vi "Coord window-Generate picture.vi"(8 "error in (no error)":errorcluster) -> (0 "error out":errorcluster)   [LabVIEW 2013]
uses:
  Globals/Coord window-Globals.vi
panel:
  in  "List":i32[](listbox)
  out "Picture":picture
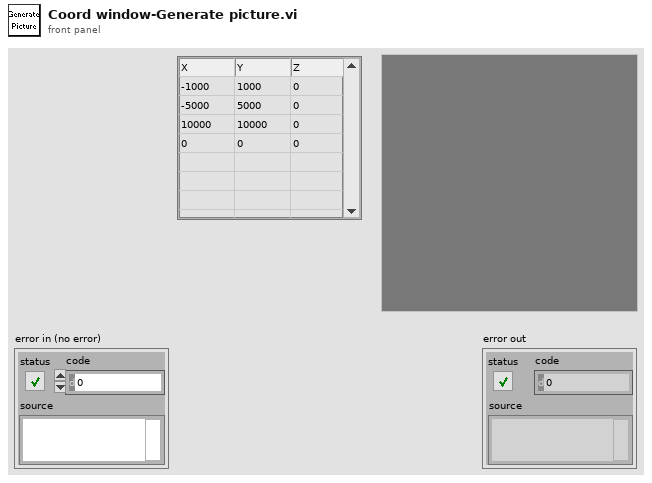
[diagram p1: front panel]
types:
  T1 = typedef "Coordinate list window refs.ctl" = cluster{"Window Name (i.e. Key)":string, "menu reference":refnum<k9>, "VI's reference":refnum<vi>, "Pane 1":refnum<vi>, "Pane 2":refnum<vi>, "Coord Listbox":refnum<vi>, "File name":refnum<vi>, "Picture Map":refnum<vi>, "Stage XYZ Position ind.":refnum<vi>}
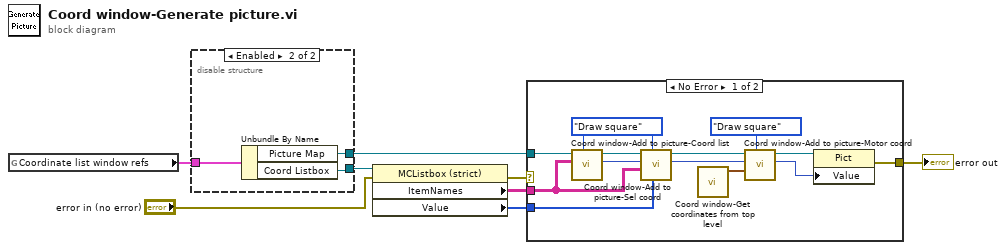
[diagram p0: block diagram]
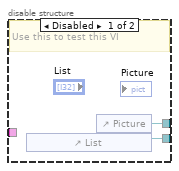
[diagram p2: hidden frame]
diagram:
  n1 = global read "Coord window-Globals.vi" "Coordinate list window refs"() -> (w2:T1)
  n2 = disable-structure "Diagram Disable Structure" shown="Enabled" {
    disable-tunnel: [w10 w11] -> w8
    disable-tunnel: [w9 w12] -> w6
    disable-tunnel: w2 -> [_ w13]
    frame Disabled {
      # "Use this to test this VI"
      n3 = control-ref of="List"() -> (w10:refnum<vi>)
      n4 = control-ref of="Picture"() -> (w9:refnum<vi>)
    }
    frame Enabled {
      n5 = Unbundle By Name(w13) -> ("Picture Map"=w12:refnum<vi>, "Coord Listbox"=w11:refnum<vi>)
    }
  }
  n6 = property on="Property Node" class="MCListbox (strict)"(reference=w8, error in="error in (no error)") -> (error out=w5:errorcluster, "ItemNames"=w7:string[][], "Value"=w4:i32[])  [unwired: 1 out]
  n7 = case shown="No Error" w5 {
    selector: w5 -> [_ w27]
    tunnel: w7 -> [w25 _]
    tunnel: w6 -> [w23 _]
    tunnel: w4 -> [w26 _]
    tunnel: [w24 w27] -> w3
    frame No Error {
      w14 = enum16{"Draw point", "Draw square"}."Draw square" ("Feature to draw")
      n8 = call "Coord window-Add to picture-Coord list.vi"("Feature to draw"=w14, "ItemNames"=w25, "Picture in"=w23) -> ("new picture"=w20:picture, "Picture out"=w17:refnum<vi>)  [unwired: 7 in]
      n9 = call "Coord window-Add to picture-Sel coord.vi"("Value"=w26, "Feature to draw"=w14, "ItemNames"=w25, "new picture in"=w20, "Picture map ref in"=w17) -> ("new picture out"=w19:picture, "Picture map ref"=w18:refnum<vi>)  [unwired: 5 in]
      n10 = call "Coord window-Get coordinates from top level.vi"() -> ("Coordinates"=w16:cluster{"X":sgl, "Y":sgl, "Z":sgl})  [unwired: 11 in]
      n11 = call "Coord window-Add to picture-Motor coord.vi"("Feature to draw"=enum16{"Draw point", "Draw square"}."Draw square", "Motor coordinates"=w16, "new picture in"=w19, "Picture in"=w18) -> ("new picture"=w22:picture, "Picture out"=w21:refnum<vi>)  [unwired: 6 in]
      n12 = property on="Property Node" class="Pict"(reference=w21, "Value"=w22) -> (error out=w24:errorcluster)  [unwired: 1 in, 1 out]
    }
    frame Error {
    }
  }
  "error out" <- w3
